vi "Practica_medicion_remota_LECTURA.vi"() -> ()   [LabVIEW 2020]
uses:
  <vilib>/httpClient/LabVIEWHTTPClient.lvlib
panel:
  in  "stop":bool
  out "Led Relé":bool
  out "Feedback [mA]":dbl
  out "Hora 2":string
  out "Hora":string
  out "Data":string
  out "error out":errorcluster
  out "body":string
  out "headers":string
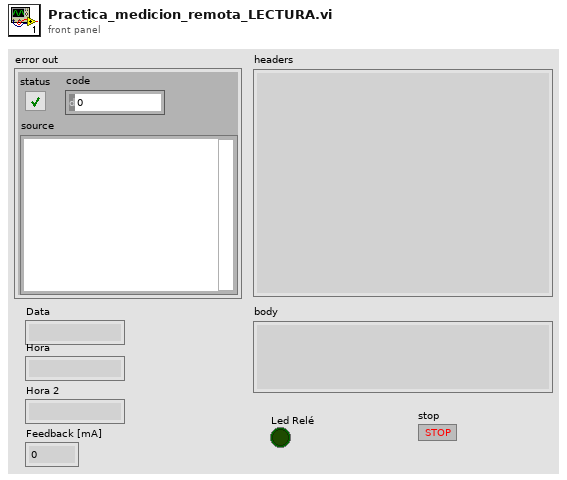
[diagram p1: front panel]
types:
  T1 = cluster{"Acondicionamiento":dbl, "Data":string, "Hora":string, "Rele":bool}
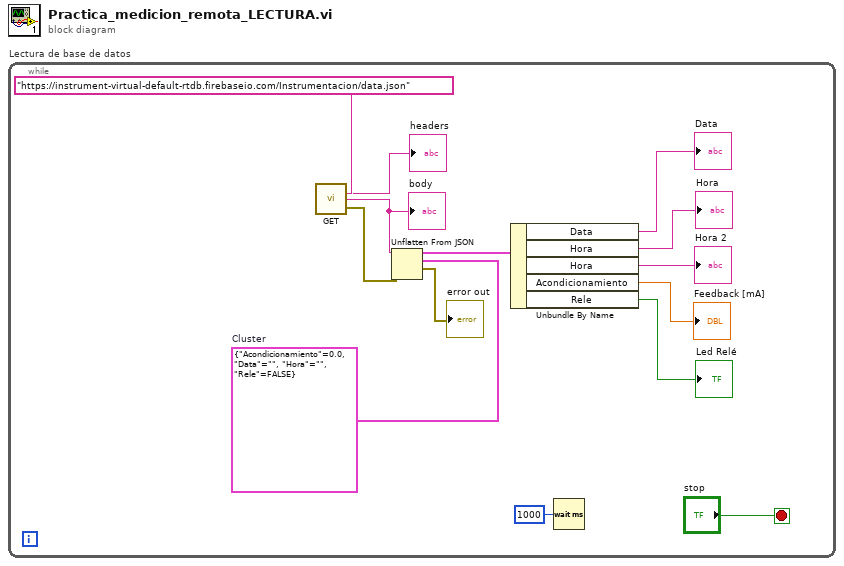
[diagram p0: block diagram]
diagram:
  n1 = while "Lectura de base de datos" {
    stop <- "stop" stop-if-true
    w10 = T1 {"Acondicionamiento"=0.0, "Data"="", "Hora"="", "Rele"=FALSE}  # Cluster
    n2 = call <vilib>:"GET.vi"("url"="https://instrument-virtual-default-rtdb.firebaseio.com/Instrumentacion/data.json") -> ("headers"=→"headers":string, "body"=w9:string, "error out"=w8:errorcluster)  [unwired: 11 in, 1 out]
    "body" <- w9
    n3 = Unflatten From JSON(JSON string=w9, type and defaults=w10, error in (no error)=w8) -> (value=w7:T1, error out=→"error out":errorcluster)  [unwired: 4 in]
    n4 = Unbundle By Name "Unbundle By Name"(w7) -> ("Data"=→"Data":string, "Hora"=→"Hora":string, "Hora"=→"Hora 2":string, "Acondicionamiento"=→"Feedback [mA]":dbl, "Rele"=→"Led Relé":bool)
    n5 = Wait (ms)(milliseconds to wait=u32 1000) -> ()  [unwired: 1 out]
  }
